vi "arrayCurFreq (SubVI).vi"(8 "Interpolation factor (n)":i32=2, 9 "Частота, Гц":dbl, 10 "ArrayFreq":dbl[](array[numeric]), 11 "ArrayIn":cluster{"X Values":dbl[], "Y Values":dbl[]}[](array[cluster])) -> (2 "ArrayFreqOut":dbl[](array[numeric]), 3 "ArrayOut":cluster{dbl[], dbl[]}[](array[cluster]))   [LabVIEW 2017]
uses:
  <vilib>/Analysis/NI_AALPro.lvlib
panel:
  in  "Type of Interpolation":T1(ring)=enum."Spline"
  out "y value":dbl
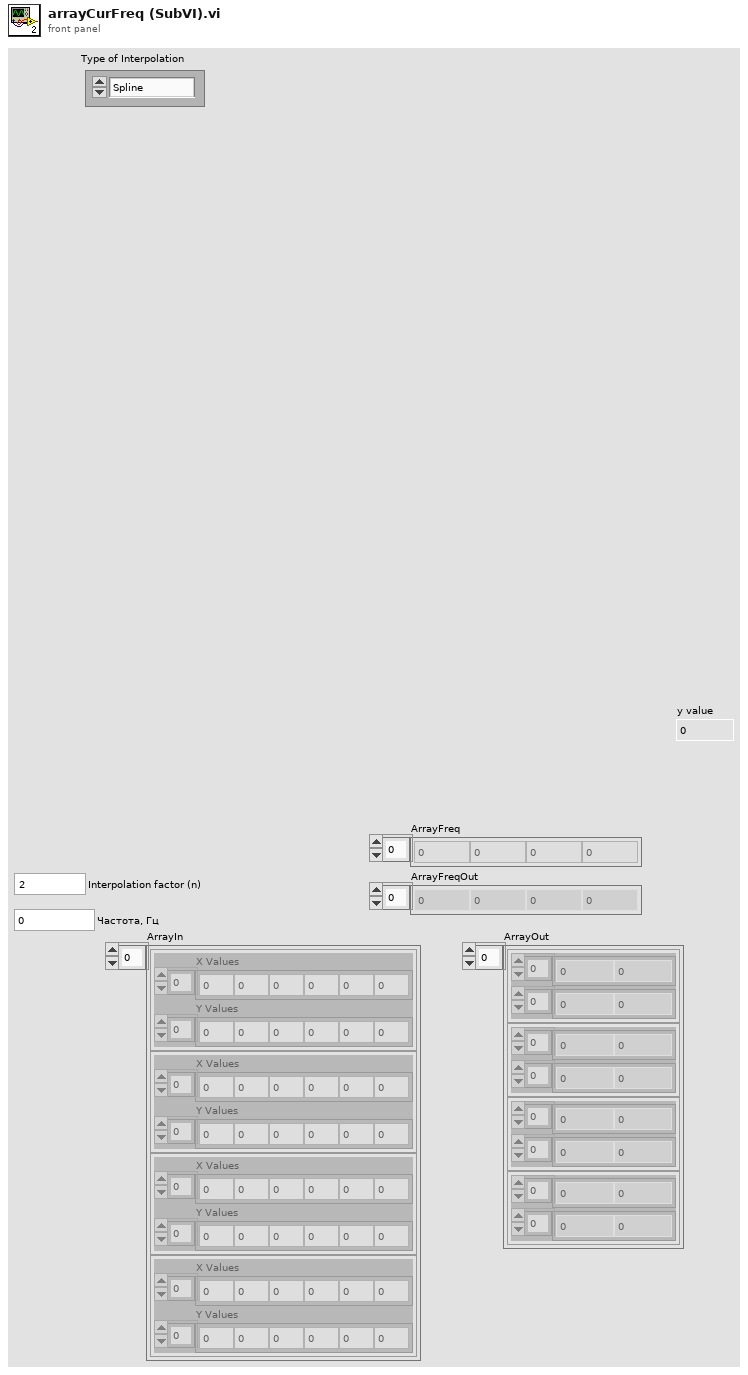
[diagram p1: front panel]
types:
  T1 = enum16{"Linear", "Polynomial", "Spline", "Rational"}
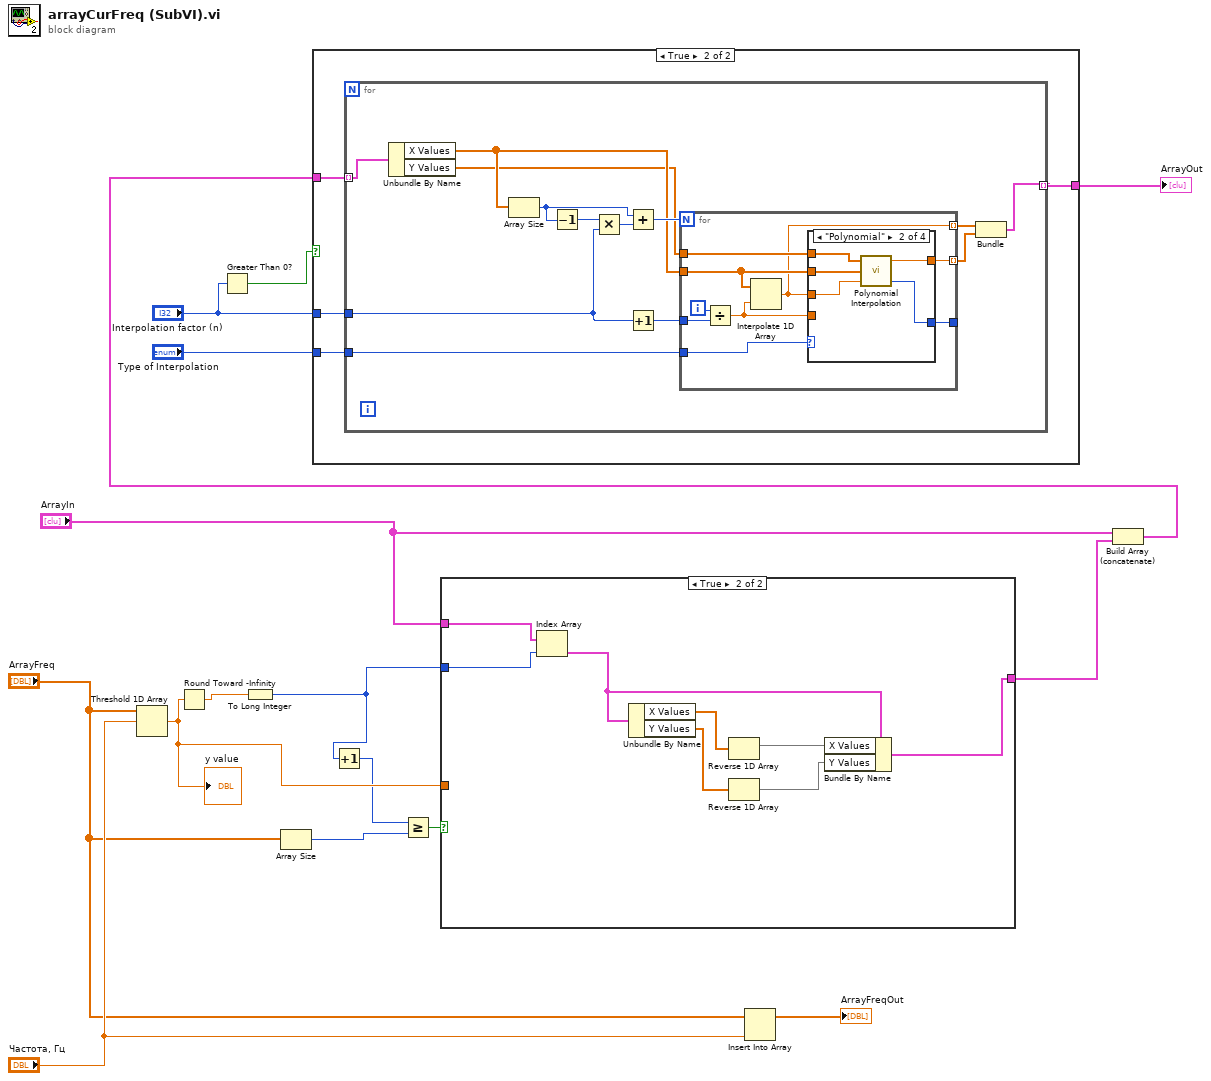
[diagram p0: block diagram]
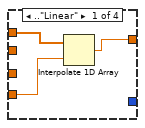
[diagram p3: hidden frame]
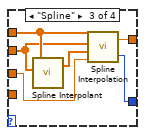
[diagram p4: hidden frame]
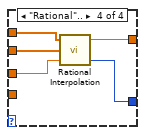
[diagram p5: hidden frame]
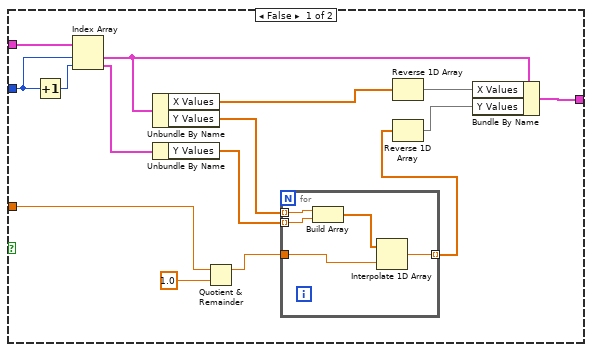
[diagram p6: hidden frame]
diagram:
  n1 = Threshold 1D Array(2:"Частота, Гц", 3:"ArrayFreq") -> (0:w16:dbl)  [unwired: 1 in]
  "y value" <- w16
  n2 = Round Toward -Infinity(1:w16) -> (0:w15:dbl)
  n3 = Greater Than 0?(x="Interpolation factor (n)") -> (x > 0?=w3:bool)
  n4 = To Long Integer(number=w15) -> (32bit integer=w2:i32)
  n5 = Array Size(array="ArrayFreq") -> (size(s)=w12:i32)
  n6 = Increment(x=w2) -> (x+1=w1:i32)
  n7 = Greater Or Equal?(x=w1, y=w12) -> (x >= y?=w11:bool)
  n8 = case shown="True" w11 {
    tunnel: w16 -> [w23 _]
    tunnel: w2 -> [w29 w43]
    tunnel: "ArrayIn" -> [w31 w44]
    tunnel: [w24 w38] -> w8
    frame False {
      n9 = Increment(x=w29) -> (x+1=w30:i32)
      n10 = Index Array(array=w31, index #1=w29, index #2=w30) -> (element #1=w25:cluster{"X Values":dbl[], "Y Values":dbl[]}, element #2=w28:cluster{"X Values":dbl[], "Y Values":dbl[]})
      n11 = Unbundle By Name(w25) -> ("X Values"=w20:dbl[], "Y Values"=w27:dbl[])
      n12 = Unbundle By Name(w28) -> ("Y Values"=w26:dbl[])
      n13 = Quotient & Remainder(x=w23, y=1.0) -> (x-y*floor(x/y)=w21:dbl)  [unwired: 1 out]
      n14 = for {
        tunnel: w27 -> [w36] mode=indexing
        tunnel: w26 -> [w35] mode=indexing
        tunnel: w21 -> [w34]
        tunnel: [w33] -> w18 mode=indexing
        n15 = Build Array(w36, w35) -> (w32:dbl[])
        n16 = Interpolate 1D Array(1:w34, 2:w32) -> (0:w33:dbl)
      }
      n17 = Reverse 1D Array(array=w20) -> (reversed array=w19:dbl[])
      n18 = Reverse 1D Array(array=w18) -> (reversed array=w17:dbl[])
      n19 = Bundle By Name(cluster=w25, "X Values"=w19, "Y Values"=w17) -> (w24:cluster{"X Values":dbl[], "Y Values":dbl[]})
    }
    frame True {
      n20 = Index Array(array=w44, index=w43) -> (element=w37:cluster{"X Values":dbl[], "Y Values":dbl[]})
      n21 = Unbundle By Name(w37) -> ("X Values"=w42:dbl[], "Y Values"=w41:dbl[])
      n22 = Reverse 1D Array(array=w42) -> (reversed array=w40:dbl[])
      n23 = Reverse 1D Array(array=w41) -> (reversed array=w39:dbl[])
      n24 = Bundle By Name(cluster=w37, "X Values"=w40, "Y Values"=w39) -> (w38:cluster{"X Values":dbl[], "Y Values":dbl[]})
    }
  }
  n25 = Insert Into Array(array="ArrayFreq", new element="Частота, Гц") -> (→"ArrayFreqOut":dbl[])  [unwired: 1 in]
  n26 = Build Array (concatenate)("ArrayIn", w8) -> (w7:cluster{"X Values":dbl[], "Y Values":dbl[]}[])
  n27 = case shown="True" w3 {
    tunnel: w7 -> [w45 w49]
    tunnel: [w45 w48] -> w6
    tunnel: "Interpolation factor (n)" -> [_ w47]
    tunnel: "Type of Interpolation" -> [_ w46]
    frame False {
    }
    frame True {
      n28 = for {
        tunnel: w49 -> [w53] mode=indexing
        tunnel: [w52] -> w48 mode=indexing
        tunnel: w47 -> [w51]
        tunnel: w46 -> [w50]
        n29 = Unbundle By Name(w53) -> ("X Values"=w55:dbl[], "Y Values"=w54:dbl[])
        n30 = Array Size(array=w55) -> (size(s)=w59:i32)
        n31 = Decrement(x=w59) -> (x-1=w62:i32)
        n32 = Multiply(x=w62, y=w51) -> (x*y=w60:i32)
        n33 = Add(x=w59, y=w60) -> (x+y=w58:i32)
        n34 = Increment(x=w51) -> (x+1=w61:i32)
        n35 = for {
          N: w58 -> [_]
          tunnel: w54 -> [w71]
          tunnel: w55 -> [w66]
          tunnel: [w70] -> _
          tunnel: w61 -> [w68]
          tunnel: [w67] -> w56 mode=indexing
          tunnel: [w65] -> w57 mode=indexing
          tunnel: w50 -> [w63]
          i -> [w69]
          n36 = Divide(x=w69, y=w68) -> (x/y=w64:dbl)
          n37 = Interpolate 1D Array(1:w64, 2:w66) -> (0:w65:dbl)
          n38 = case shown="\"Polynomial\"" w63 {
            tunnel: w65 -> [_ w79 w82 w86]
            tunnel: [w73 w78 w80 w88] -> w67
            tunnel: [_ w77 w81 w87] -> w70
            tunnel: w66 -> [_ w76 w83 w89]
            tunnel: w71 -> [w74 w75 w85 w90]
            tunnel: w64 -> [w72 _ _ _]
            frame .."Linear" {
              n39 = Interpolate 1D Array(1:w72, 2:w74) -> (0:w73:dbl)
            }
            frame "Polynomial" {
              n40 = call <vilib>:"Polynomial Interpolation.vi"("x value"=w79, "X"=w76, "Y"=w75) -> ("error"=w77:i32, "interpolation value"=w78:dbl)  [unwired: 1 out]
            }
            frame "Spline" {
              n41 = call <vilib>:"Spline Interpolant.vi"("X"=w83, "Y"=w85) -> ("Interpolant"=w84:dbl[])  [unwired: 2 in, 1 out]
              n42 = call <vilib>:"Spline Interpolation.vi"("x value"=w82, "Interpolant"=w84, "X"=w83, "Y"=w85) -> ("error"=w81:i32, "interpolation value"=w80:dbl)
            }
            frame "Rational".. {
              n43 = call <vilib>:"Rational Interpolation.vi"("x value"=w86, "X"=w89, "Y"=w90) -> ("error"=w87:i32, "interpolation value"=w88:dbl)  [unwired: 1 out]
            }
          }
        }
        n44 = Bundle(w57, w56) -> (w52:cluster{dbl[], dbl[]})  [unwired: 1 in]
      }
    }
  }
  "ArrayOut" <- w6
